vi "Binary Streaming Instrument.vi"() -> ()   [LabVIEW 2019]
uses:
  <vilib>/Instr/_visa.llb/VISA Configure Serial Port (Instr).vi
panel:
  out "Max & Min":dbl[](array[numeric])
  out "error out":errorcluster
  in  "stop":bool
  in  "VISA resource name":refnum<visa-resource-name>
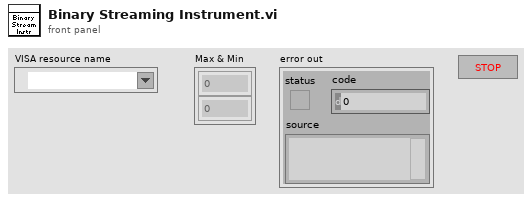
[diagram p1: front panel]
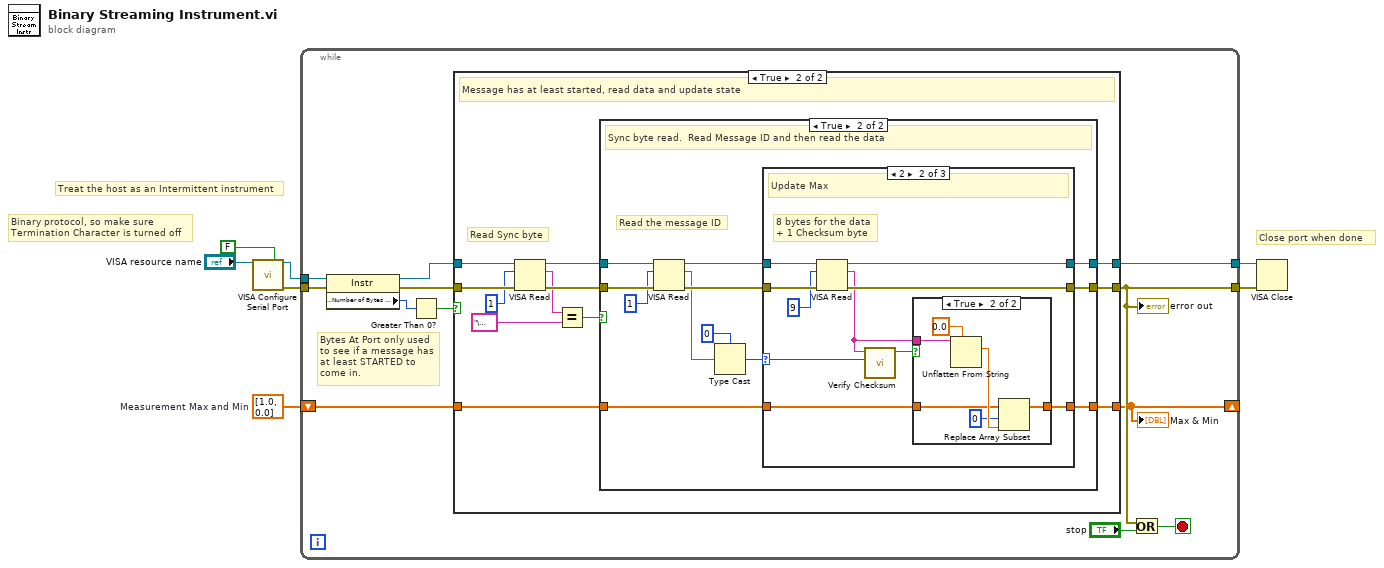
[diagram p0: block diagram]
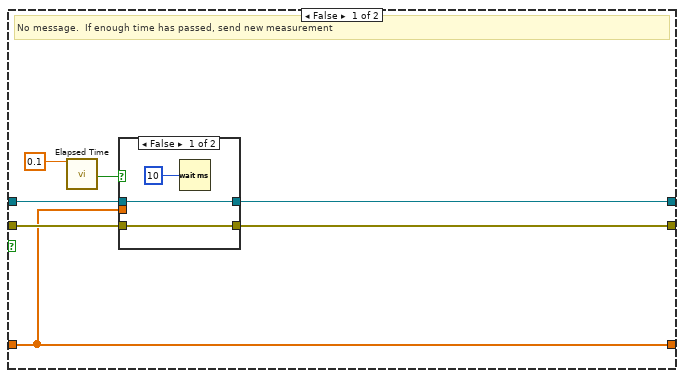
[diagram p2: hidden frame]
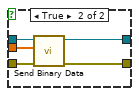
[diagram p3: hidden frame]
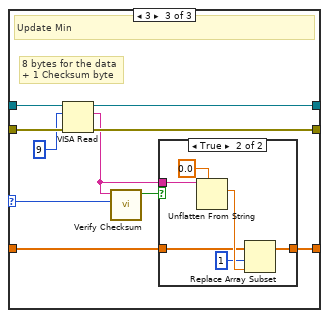
[diagram p7: hidden frame]
diagram:
  w3 = dbl[] [1.0, 0.0]  # Measurement Max and Min
  # "Binary protocol, so make sure\nTermination Character is turned off"
  # "Treat the host as an Intermittent instrument"
  # "Close port when done"
  n1 = call-poly "VISA Configure Serial Port"("VISA resource name"="VISA resource name", "Enable Termination\nChar (T)"=FALSE ("Enable Termination\nChar (T)")) -> ("VISA resource name out"=w2:refnum<visa-resource-name>, "error out"=w6:errorcluster)  [unwired: 12 in]
  n2 = while {
    tunnel: w6 -> [w19]
    tunnel: w2 -> [w16]
    tunnel: [w12] -> w4
    tunnel: [w17] -> w7
    shift-right: [w8] -> _
    shift-left: w3 -> [w9]
    stop <- w11 stop-if-true
    # "Bytes At Port only used\nto see if a message has\nat least STARTED to\ncome in."
    n3 = property class="Instr"(reference=w16, error in=w19) -> (reference out=w13:refnum<visa-resource-name>, error out=w18:errorcluster, "Serial Settings:Number of Bytes at Serial Port"=w15:u32)
    n4 = Greater Than 0?(x=w15) -> (x > 0?=w14:bool)
    n5 = case shown="True" w14 {
      tunnel: w18 -> [w26 w46]
      tunnel: w13 -> [w23 w43]
      tunnel: [w20 w35] -> w12
      tunnel: [w25 w44] -> w17
      tunnel: w9 -> [w21 w37]
      tunnel: [w21 w36] -> w8
      frame False {
        # "No message.  If enough time has passed, send new measurement"
        n6 = call "Elapsed Time"("Time Target (s)"=0.1) -> ("Time has Elapsed"=w22:bool)  [unwired: 11 in, 7 out]
        n7 = case shown="False" w22 {
          tunnel: w23 -> [w28 w32]
          tunnel: w26 -> [w29 w34]
          tunnel: w21 -> [_ w30]
          tunnel: [w28 w31] -> w20
          tunnel: [w29 w33] -> w25
          frame False {
            n8 = Wait (ms)(milliseconds to wait=u32 10) -> ()  [unwired: 1 out]
          }
          frame True {
            n9 = call "Send Binary Data.vi"("error in"=w34, "Measurement Max and Min"=w30, "VISA Refnum in"=w32) -> ("error out"=w33:errorcluster, "VISA Refnum out"=w31:refnum<visa-resource-name>)  [unwired: 7 in]
          }
        }
      }
      frame True {
        # "Read Sync byte"
        # "Message has at least started, read data and update state"
        n10 = VISA Read(VISA resource name=w43, byte count=u32 1, error in (no error)=w46) -> (VISA resource name out=w39:refnum<visa-resource-name>, read buffer=w38:string, error out=w45:errorcluster)  [unwired: 1 out]
        n11 = Equal?(x=w38, y="\u0002") -> (x = y?=w40:bool)
        n12 = case shown="True" w40 {
          tunnel: w39 -> [w48 w57]
          tunnel: w45 -> [w49 w61]
          tunnel: [w48 w52] -> w35
          tunnel: [w49 w59] -> w44
          tunnel: w37 -> [w47 w51]
          tunnel: [w47 w50] -> w36
          frame False {
            # "Sync byte was not read.  Ignore the data assuming we are in the middle of a message."
          }
          frame True {
            # "Read the message ID"
            # "Sync byte read.  Read Message ID and then read the data"
            n13 = VISA Read(VISA resource name=w57, byte count=u32 1, error in (no error)=w61) -> (VISA resource name out=w53:refnum<visa-resource-name>, read buffer=w56:string, error out=w60:errorcluster)  [unwired: 1 out]
            n14 = Type Cast(type=u8 0, x=w56) -> (*(type *) &x=w54:u8)
            n15 = case shown="2" w54 {
              selector: w54 -> [_ w68 w85]
              tunnel: w60 -> [w64 w74 w91]
              tunnel: w53 -> [w63 w72 w89]
              tunnel: [w63 w70 w87] -> w52
              tunnel: [w64 w73 w90] -> w59
              tunnel: w51 -> [w62 w66 w83]
              tunnel: [w62 w65 w82] -> w50
              frame Default {
                # "Unknown ID.  Ignore the data"
              }
              frame 2 {
                # "8 bytes for the data\n+ 1 Checksum byte"
                # "Update Max"
                n16 = VISA Read(VISA resource name=w72, byte count=u32 9, error in (no error)=w74) -> (VISA resource name out=w70:refnum<visa-resource-name>, read buffer=w67:string, error out=w73:errorcluster)  [unwired: 1 out]
                n17 = call "Verify Checksum.vi"("Message ID"=w68, "Data + Checksum"=w67) -> ("Pass"=w69:bool)  [unwired: 9 in]
                n18 = case shown="True" w69 {
                  tunnel: w67 -> [_ w80]
                  tunnel: w66 -> [w75 w77]
                  tunnel: [w75 w76] -> w65
                  frame False {
                  }
                  frame True {
                    n19 = Unflatten From String(type=0.0, binary string=w80) -> (value=w81:dbl)  [unwired: 3 in, 2 out]
                    n20 = Replace Array Subset(array=w77, new element=w81, index=0) -> (w76:dbl[])
                  }
                }
              }
              frame 3 {
                # "8 bytes for the data\n+ 1 Checksum byte"
                # "Update Min"
                n21 = VISA Read(VISA resource name=w89, byte count=u32 9, error in (no error)=w91) -> (VISA resource name out=w87:refnum<visa-resource-name>, read buffer=w84:string, error out=w90:errorcluster)  [unwired: 1 out]
                n22 = call "Verify Checksum.vi"("Message ID"=w85, "Data + Checksum"=w84) -> ("Pass"=w86:bool)  [unwired: 9 in]
                n23 = case shown="True" w86 {
                  tunnel: w84 -> [_ w97]
                  tunnel: w83 -> [w92 w94]
                  tunnel: [w92 w93] -> w82
                  frame False {
                  }
                  frame True {
                    n24 = Unflatten From String(type=0.0, binary string=w97) -> (value=w98:dbl)  [unwired: 3 in, 2 out]
                    n25 = Replace Array Subset(array=w94, new element=w98, index=1) -> (w93:dbl[])
                  }
                }
              }
            }
          }
        }
      }
    }
    "error out" <- w17
    "Max & Min" <- w8
    n26 = Or(x=w17, y="stop") -> (x .or. y?=w11:bool)
  }
  n27 = VISA Close(VISA resource name=w4, error in (no error)=w7) -> ()  [unwired: 1 out]
